vi "64 to 8 Bit Cluster (SubVI).vi"(11 "Data In":u64) -> (3 "Data Out":T1)   [LabVIEW 2015]
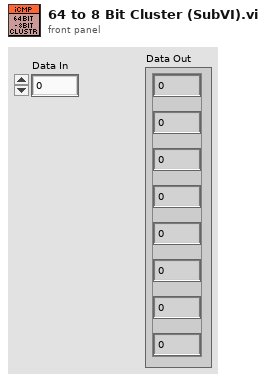
[diagram p1: front panel]
types:
  T1 = cluster{"Numeric Control":u8, "Numeric Control":u8, "Numeric Control":u8, "Numeric Control":u8, "Numeric Control":u8, "Numeric Control":u8, "Numeric Control":u8, "Numeric Control":u8}
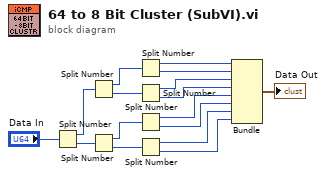
[diagram p0: block diagram]
diagram:
  n1 = Split Number(x="Data In") -> (hi(x)=w11:u32, lo(x)=w10:u32)
  n2 = Split Number(x=w11) -> (hi(x)=w15:u16, lo(x)=w14:u16)
  n3 = Split Number(x=w10) -> (hi(x)=w13:u16, lo(x)=w12:u16)
  n4 = Split Number(x=w15) -> (hi(x)=w9:u8, lo(x)=w7:u8)
  n5 = Split Number(x=w14) -> (hi(x)=w6:u8, lo(x)=w5:u8)
  n6 = Split Number(x=w13) -> (hi(x)=w4:u8, lo(x)=w3:u8)
  n7 = Split Number(x=w12) -> (hi(x)=w2:u8, lo(x)=w1:u8)
  n8 = Bundle(w9, w7, w6, w5, w4, w3, w2, w1) -> (→"Data Out":cluster{u8, u8, u8, u8, u8, u8, u8, u8})  [unwired: 1 in]
